vi "Check BaseNodeTypes Deep Equal.vi"(8 "error in (no error)":errorcluster, 9 "Settings":T1, 10 "BaseNodeType 2":refnum<k24>, 11 "BaseNodeType 1":refnum<k24>) -> (0 "error out":errorcluster, 1 "Equal?":bool, 2 "BaseNodeType 2":refnum<k24>, 3 "BaseNodeType 1":refnum<k24>, 4 "Inequality context":string)   [LabVIEW 2017, in "SLSC Switch Import Export Unit Tests.lvclass"]
uses:
  SLSC Switch Import Export Unit Tests.lvclass
  NationalInstruments.VeriStand.SystemStorage
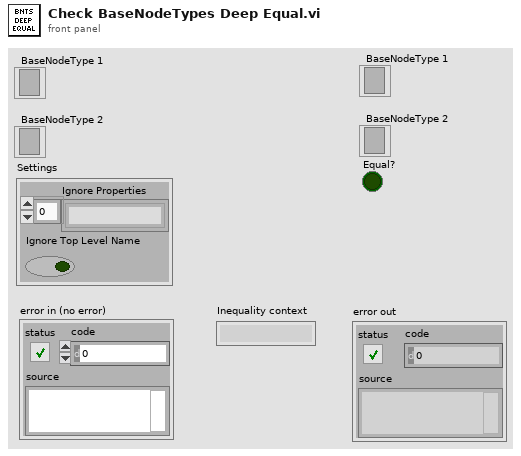
[diagram p1: front panel]
types:
  T1 = cluster{"Ignore Properties":string[], "Ignore Top Level Name":bool}
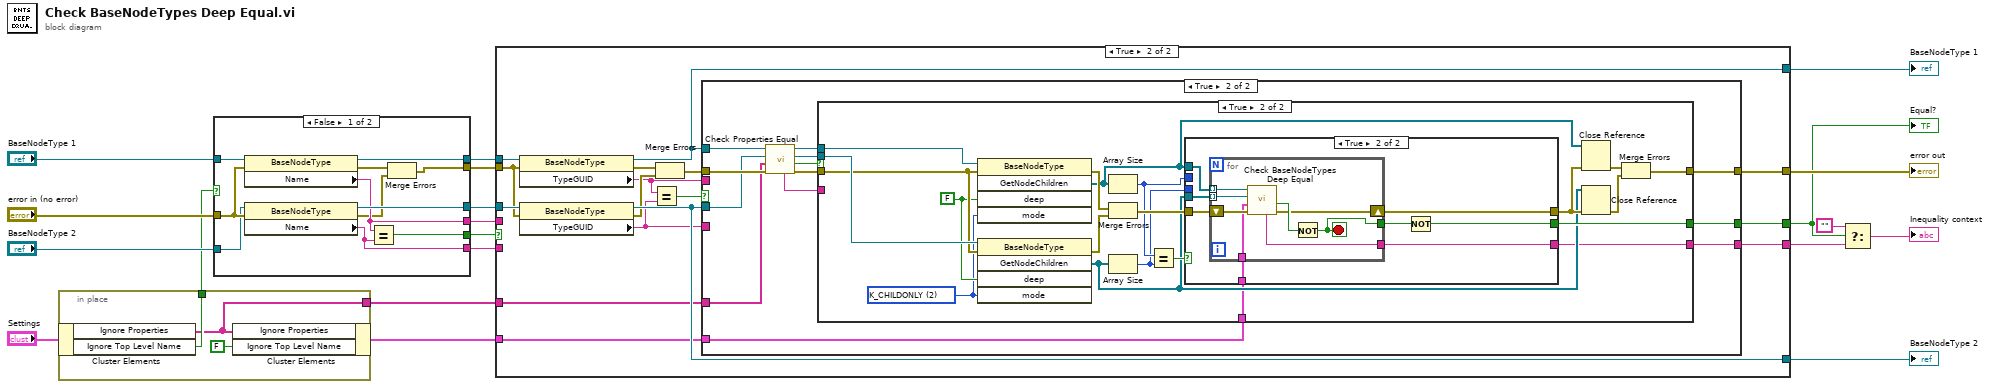
[diagram p0: block diagram]
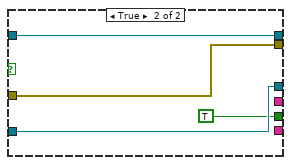
[diagram p2: hidden frame]
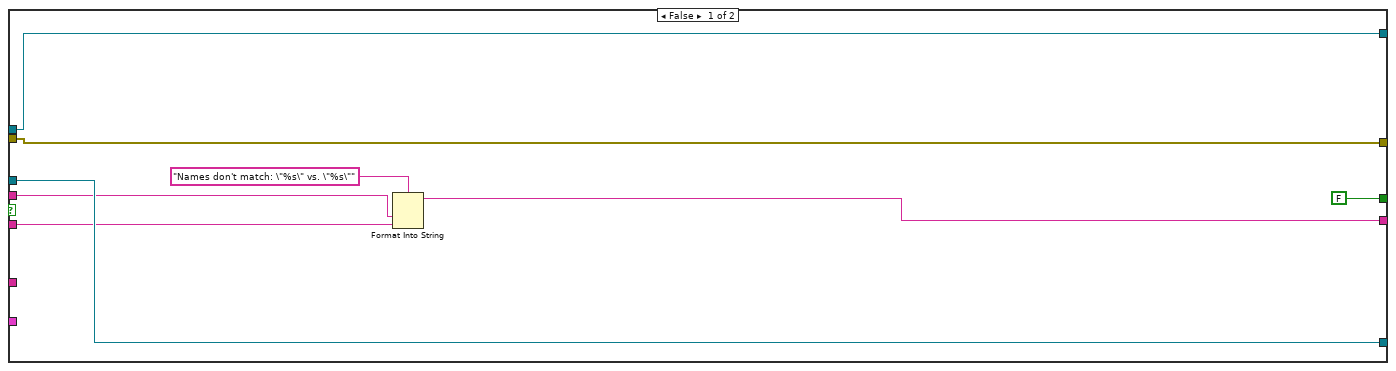
[diagram p3: hidden frame]
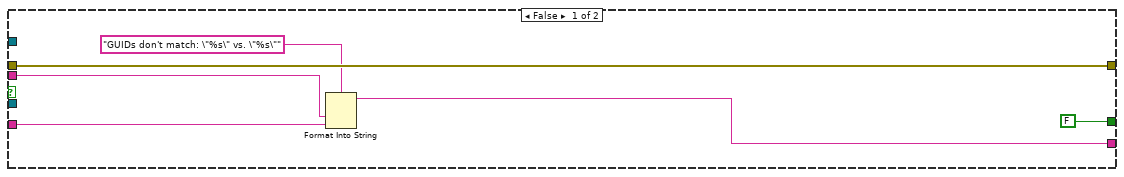
[diagram p4: hidden frame]
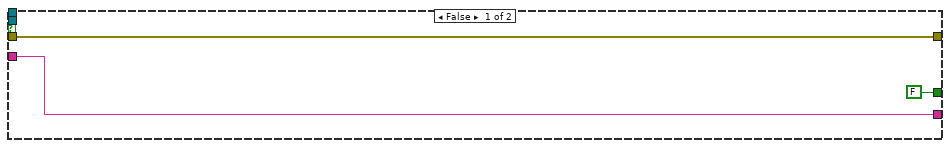
[diagram p5: hidden frame]
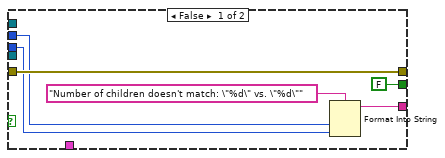
[diagram p6: hidden frame]
diagram:
  n1 = in-place {
    in-place-border: [w22] -> w3
    in-place-border: [w21] -> w1
    n2 = in-place-cluster #1("Settings") -> ("Ignore Properties"=w21:string[], "Ignore Top Level Name"=w22:bool)
    n3 = in-place-cluster #1("Ignore Properties"=w21, "Ignore Top Level Name"=FALSE) -> (w2:T1)
  }
  n4 = case shown="False" w3 {
    tunnel: "error in (no error)" -> [w34 w38]
    tunnel: "BaseNodeType 2" -> [w33 w36]
    tunnel: "BaseNodeType 1" -> [w32 w37]
    tunnel: [w31 w37] -> w16
    tunnel: [w30 w36] -> w15
    tunnel: [w25 w38] -> w12
    tunnel: [w28 TRUE] -> w11
    tunnel: [w27 _] -> w10
    tunnel: [w26 _] -> w9
    frame False {
      n5 = property class="BaseNodeType"(reference=w32, error in=w34) -> (reference out=w31:refnum<k24>, error out=w29:errorcluster, "Name"=w27:string)
      n6 = property class="BaseNodeType"(reference=w33, error in=w34) -> (reference out=w30:refnum<k24>, error out=w24:errorcluster, "Name"=w26:string)
      n7 = Equal?(x=w27, y=w26) -> (x = y?=w28:bool)
      n8 = Merge Errors(w29, w24) -> (w25:errorcluster)
    }
    frame True {
    }
  }
  n9 = case shown="True" w11 {
    tunnel: [FALSE w61] -> w8
    tunnel: [w46 w60] -> w17
    tunnel: w16 -> [w45 w59]
    tunnel: w15 -> [w44 w58]
    tunnel: [w44 w57] -> w14
    tunnel: [w45 w56] -> w13
    tunnel: w12 -> [w46 w47]
    tunnel: w10 -> [w42 _]
    tunnel: w9 -> [w41 _]
    tunnel: [w40 w50] -> w7
    tunnel: w2 -> [_ w49]
    tunnel: w1 -> [_ w48]
    frame False {
      n10 = Format Into String(format string="Names don't match: \"%s\" vs. \"%s\"", w42, w41) -> (resulting string=w40:string)  [unwired: 2 in, 1 out]
    }
    frame True {
      n11 = property class="BaseNodeType"(reference=w59, error in=w47) -> (reference out=w56:refnum<k24>, error out=w55:errorcluster, "TypeGUID"=w52:string)
      n12 = property class="BaseNodeType"(reference=w58, error in=w47) -> (reference out=w57:refnum<k24>, error out=w54:errorcluster, "TypeGUID"=w51:string)
      n13 = Equal?(x=w52, y=w51) -> (x = y?=w53:bool)
      n14 = Merge Errors(w55, w54) -> (w62:errorcluster)
      n15 = case shown="True" w53 {
        tunnel: w62 -> [w67 w77]
        tunnel: [FALSE w76] -> w61
        tunnel: [w67 w75] -> w60
        tunnel: w57 -> [_ w74]
        tunnel: w56 -> [_ w73]
        tunnel: w52 -> [w65 _]
        tunnel: w51 -> [w64 _]
        tunnel: [w63 w72] -> w50
        tunnel: w49 -> [_ w70]
        tunnel: w48 -> [_ w69]
        frame False {
          n16 = Format Into String(format string="GUIDs don't match: \"%s\" vs. \"%s\"", w65, w64) -> (resulting string=w63:string)  [unwired: 2 in, 1 out]
        }
        frame True {
          n17 = call "Check Properties Equal.vi"("error in"=w77, "Ignore Properties"=w69, "BaseNodeType 2"=w74, "BaseNodeType 1"=w73) -> ("error out"=w79:errorcluster, "Equal?"=w81:bool, "BaseNodeType 2"=w78:refnum<k24>, "BaseNodeType 1"=w80:refnum<k24>, "Inequality context"=w71:string)  [unwired: 3 in]
          n18 = case shown="True" w81 {
            tunnel: w78 -> [_ w104]
            tunnel: w79 -> [w83 w103]
            tunnel: w80 -> [_ w102]
            tunnel: [FALSE w98] -> w76
            tunnel: [w83 w92] -> w75
            tunnel: [w82 w88] -> w72
            tunnel: w71 -> [w82 _]
            tunnel: w70 -> [_ w85]
            frame False {
            }
            frame True {
              w100 = 2 items=["K_BFS", "K_DFS", "K_CHILDONLY", "K_UP"] ("mode")
              w101 = FALSE ("deep")
              n19 = invoke class="BaseNodeType" method="GetNodeChildren"(reference=w102, error in=w103, "deep"=w101, "mode"=w100) -> (error out=w97:errorcluster, "GetNodeChildren"=w90:refnum<k24>[])  [unwired: 1 in, 3 out]
              n20 = invoke class="BaseNodeType" method="GetNodeChildren"(reference=w104, error in=w103, "deep"=w101, "mode"=w100) -> (error out=w96:errorcluster, "GetNodeChildren"=w89:refnum<k24>[])  [unwired: 1 in, 3 out]
              n21 = Array Size(array=w90) -> (size(s)=w87:i32)
              n22 = Merge Errors(w97, w96) -> (w95:errorcluster)
              n23 = Array Size(array=w89) -> (size(s)=w86:i32)
              n24 = Equal?(x=w87, y=w86) -> (x = y?=w99:bool)
              n25 = case shown="True" w99 {
                tunnel: w90 -> [_ w118]
                tunnel: w89 -> [_ w117]
                tunnel: [FALSE w115] -> w98
                tunnel: w95 -> [w109 w114]
                tunnel: [w109 w113] -> w93
                tunnel: [w105 w112] -> w88
                tunnel: w87 -> [w107 _]
                tunnel: w86 -> [w106 _]
                tunnel: w85 -> [_ w111]
                frame False {
                  n26 = Format Into String(format string="Number of children doesn't match: \"%d\" vs. \"%d\"", w107, w106) -> (resulting string=w105:string)  [unwired: 2 in, 1 out]
                }
                frame True {
                  n27 = for {
                    tunnel: w118 -> [w126] mode=indexing
                    tunnel: w117 -> [w125] mode=indexing
                    tunnel: [w123] -> w116
                    shift-right: [w121] -> w113
                    shift-left: w114 -> [w122]
                    tunnel: [w120] -> w112
                    tunnel: w111 -> [w119]
                    stop <- w123 stop-if-true
                    n28 = call "Check BaseNodeTypes Deep Equal.vi"("error in (no error)"=w122, "Settings"=w119, "BaseNodeType 2"=w125, "BaseNodeType 1"=w126) -> ("error out"=w121:errorcluster, "Equal?"=w124:bool, "Inequality context"=w120:string)  [unwired: 3 in, 2 out]
                    n29 = Not(x=w124) -> (.not. x?=w123:bool)
                  }
                  n30 = Not(x=w116) -> (.not. x?=w115:bool)
                }
              }
              n31 = Close Reference(reference=w90, error in (no error)=w93) -> (error out=w94:errorcluster)
              n32 = Close Reference(reference=w89, error in (no error)=w93) -> (error out=w91:errorcluster)
              n33 = Merge Errors(w94, w91) -> (w92:errorcluster)
            }
          }
        }
      }
    }
  }
  "Equal?" <- w8
  "BaseNodeType 1" <- w13
  "BaseNodeType 2" <- w14
  "error out" <- w17
  n34 = Select(t="", s=w8, f=w7) -> (s? t:f=→"Inequality context":string)
